vi "Read alarm XML.vi"(11 "模块名称":string) -> (3 "报警输出":string[][](array[string]))   [LabVIEW 2016, in "斯坦道CODMn.lvlib"]
uses:
  <vilib>/Utility/xml.llb/Write to XML File(string).vi
  <vilib>/Utility/xml.llb/Read From XML File(string).vi
panel:
  in  "报警常量":string[][](array[string])=[["1", "1999", "电极异常", "1.ORP电极线路连接异常\n2.ORP传感器故障\n3.采集ORP的PLC模拟量采集模块故障"], ["2", "1999", "温控器故障", "1.PT100线路连接异常\n2.PT100传感器故障\n3.采集温度的PLC模拟量采集模块故障"], ["3", "2009", "加热故障", "1.PT100线路连接异常\n2.PT100传感器故障\n3.采集温度的PLC模拟量采集模块故障\n1.缺水样导致\n2.PT100异常"], ["4", "1999", "高锰酸钾异常", "1.缺高锰酸钾试剂\n2.检测水样浓度过高"], ["5", "1999", "草酸钠异常", "1.缺草酸钠试剂\n2.高锰酸钾配制浓度错误"], ["6", "1999", "测量错误", "1.检查其他异常告警"], ["7", "1999", "校标错误", "1.检查其他异常告警"], ["8", "1999", "进水样超量程", "1.进水样超过最大体积"], ["9", "1999", "排液阀故障", "1.检查排液阀\n2.检查排液管上的液位传感器"], ["10", "1999", "60分钟超时报警", "1.水样浓度过高导致超时\n2.反滴定速度过慢导致超时"], ["11", "1999", "进样无液体报警", "1.检查进样泵\n2.检查进样管上的液位传感器"]]
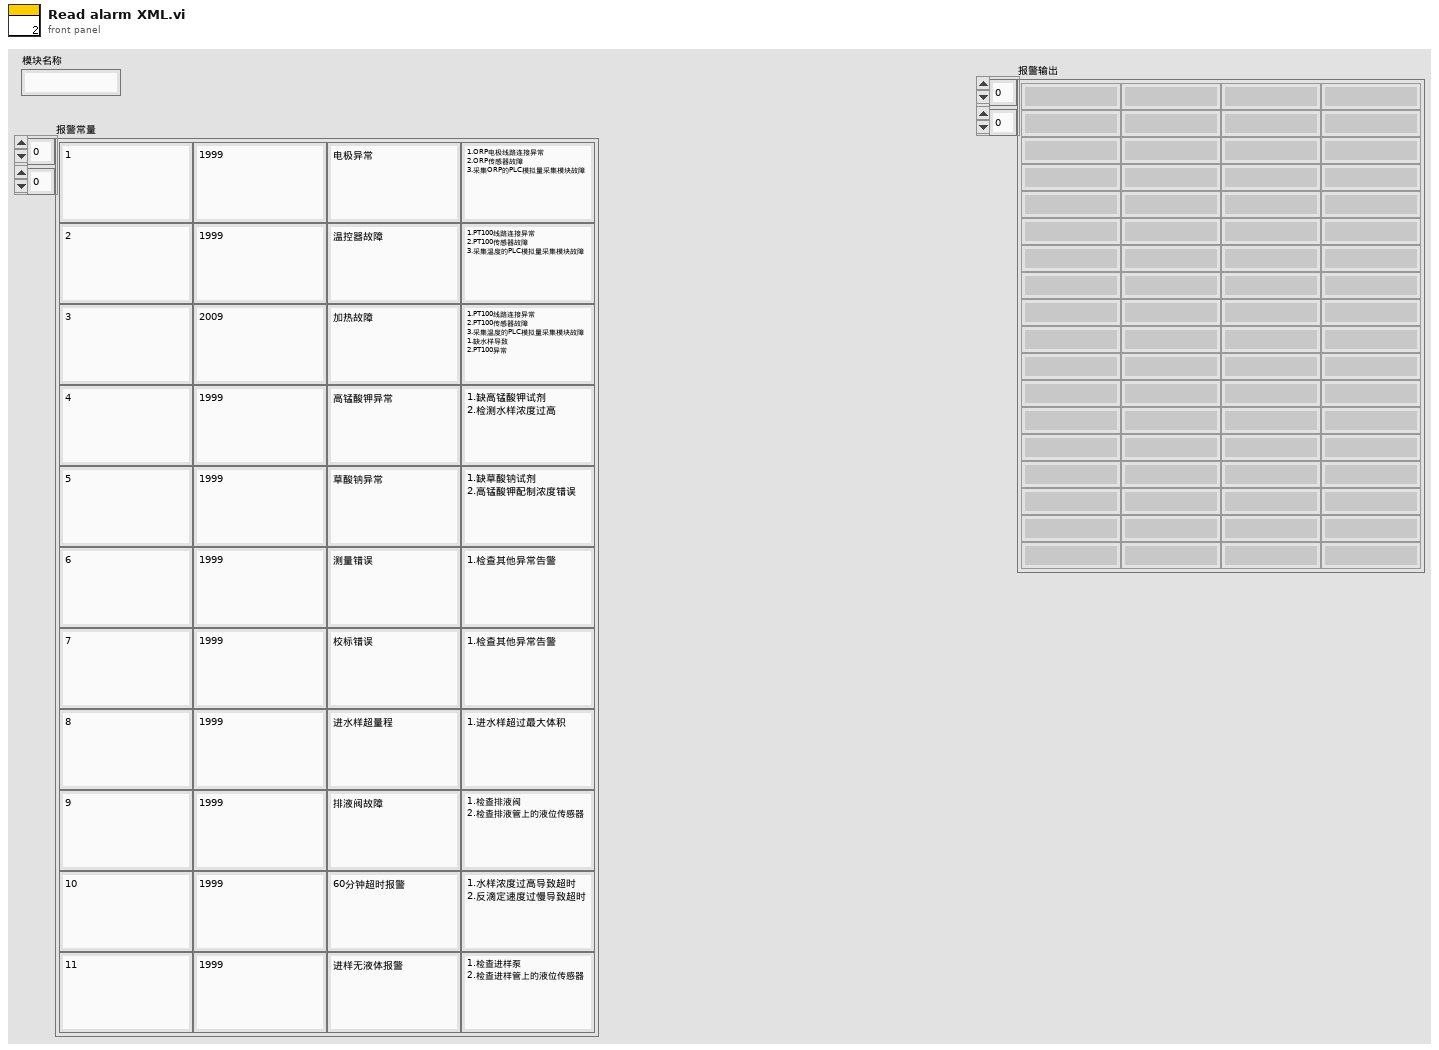
[diagram p1: front panel]
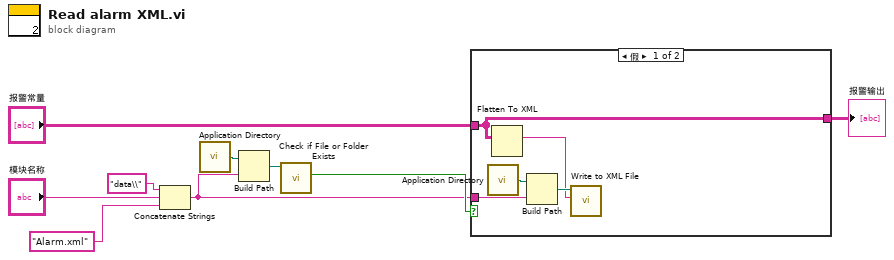
[diagram p0: block diagram]
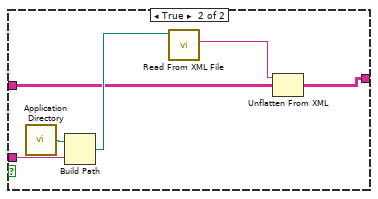
[diagram p2: hidden frame]
diagram:
  n1 = Concatenate Strings("data\\" ("字符串"), "模块名称", "Alarm.xml" ("名称或相对路径")) -> (w6:string)
  n2 = call <vilib>:"Application Directory.vi"() -> ("Application Directory"=w4:path)
  n3 = Build Path(base path=w4, name or relative path=w6) -> (appended path=w5:path)
  n4 = call <vilib>:"Check if File or Folder Exists.vi"("path"=w5) -> ("file or folder exists?"=w7:bool)  [unwired: 8 in, 2 out]
  n5 = case shown="假" w7 {
    tunnel: [w10 w17] -> w8
    tunnel: w6 -> [w11 w16]
    tunnel: "报警常量" -> [w10 w15]
    frame False {
      n6 = call <vilib>:"Application Directory.vi"() -> ("Application Directory"=w13:path)
      n7 = Flatten To XML(anything=w10) -> (xml string=w12:string)
      n8 = Build Path(base path=w13, name or relative path=w11) -> (appended path=w14:path)
      n9 = call-poly <vilib>:"Write to XML File.vi"("XML Input"=w12, "XML File Path"=w14) -> ()  [unwired: 7 in, 3 out]
    }
    frame True {
      n10 = call <vilib>:"Application Directory.vi"() -> ("Application Directory"=w19:path)
      n11 = Build Path(base path=w19, name or relative path=w16) -> (appended path=w18:path)
      n12 = call-poly <vilib>:"Read From XML File.vi"("XML File Path"=w18) -> ("XML Elements"=w20:string)  [unwired: 8 in, 2 out]
      n13 = Unflatten From XML(xml string=w20, type=w15) -> (value=w17:string[][])  [unwired: 1 in, 1 out]
    }
  }
  "报警输出" <- w8
